vi "test control disable.vi"(0 "Robot Mode":T3(ring), 1 "Test Mode":T2(ring)) -> (2 "Display Test?":bool, 3 "Why Disabled?":string, 4 "Disabled":T1(ring))   [LabVIEW 2015]
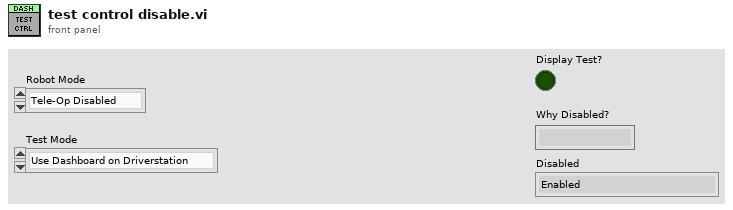
[diagram p1: front panel]
types:
  T1 = enum8{"Enabled", "Disabled", "Disabled and Grayed Out"}
  T2 = enum32{"Use Dashboard on Driverstation", "Use Programmer's Laptop"}
  T3 = enum8{"Tele-Op Disabled", "Tele-Op Enabled", "Auto Disabled", "Auto Enabled", "Test Disabled", "Test Enabled", "Disconnected", "No Code", "E-Stop"}
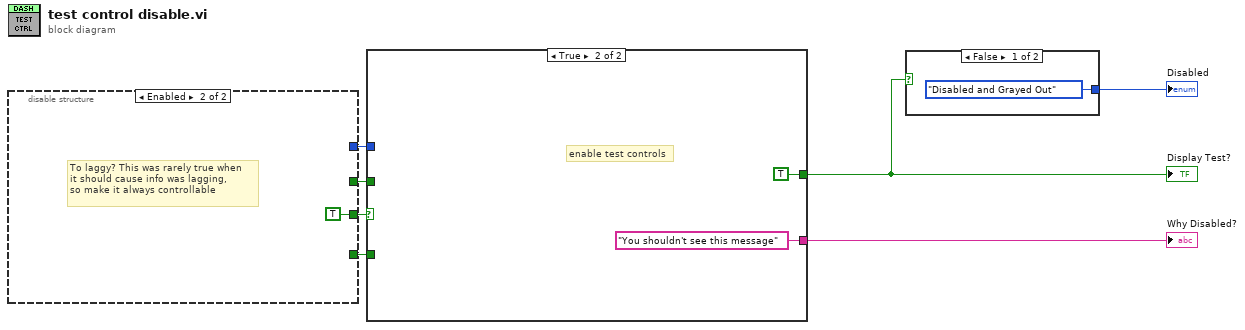
[diagram p0: block diagram]
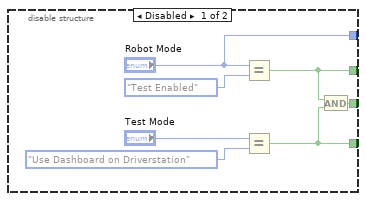
[diagram p2: hidden frame]
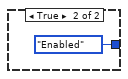
[diagram p3: hidden frame]
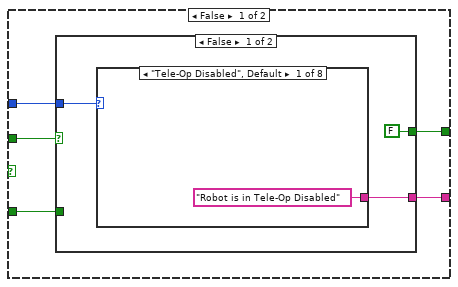
[diagram p4: hidden frame]
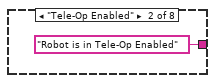
[diagram p5: hidden frame]
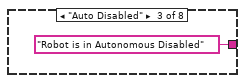
[diagram p6: hidden frame]
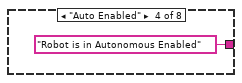
[diagram p7: hidden frame]
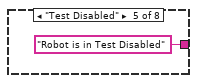
[diagram p8: hidden frame]
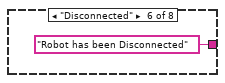
[diagram p9: hidden frame]
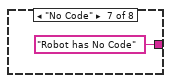
[diagram p10: hidden frame]
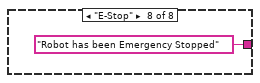
[diagram p11: hidden frame]
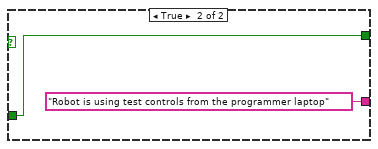
[diagram p12: hidden frame]
diagram:
  n1 = disable-structure shown="Enabled" {
    disable-tunnel: [w11 TRUE] -> w7
    disable-tunnel: [w10 _] -> w5
    disable-tunnel: [w9 _] -> w4
    disable-tunnel: ["Robot Mode" _] -> w3
    frame Disabled {
      n2 = Equal?(x="Robot Mode", y=T3."Test Enabled") -> (x = y?=w10:bool)
      n3 = Equal?(x="Test Mode", y=T2."Use Dashboard on Driverstation") -> (x = y?=w9:bool)
      n4 = And(x=w10, y=w9) -> (x .and. y?=w11:bool)
    }
    frame Enabled {
      # "To laggy? This was rarely true when\nit should cause info was lagging,\nso make it always controllable"
    }
  }
  n5 = case shown="True" w7 {
    tunnel: [w18 TRUE] -> w2
    tunnel: [w17 "You shouldn't see this message" ("Why Disabled?")] -> w6
    tunnel: w5 -> [w20 _]
    tunnel: w4 -> [w19 _]
    tunnel: w3 -> [w16 _]
    frame False {
      n6 = case shown="False" w20 {
        tunnel: w19 -> [_ w32]
        tunnel: [FALSE w32] -> w18
        tunnel: [w21 "Robot is using test controls from the programmer laptop" ("Why Disabled?")] -> w17
        tunnel: w16 -> [w22 _]
        frame False {
          n7 = case shown="\"Tele-Op Disabled\", Default" w22 {
            tunnel: ["Robot is in Tele-Op Disabled" ("Why Disabled?") "Robot is in Tele-Op Enabled" ("Why Disabled?") "Robot is in Autonomous Disabled" ("Why Disabled?") "Robot is in Autonomous Enabled" ("Why Disabled?") "Robot is in Test Disabled" ("Why Disabled?") "Robot has been Disconnected" ("Why Disabled?") "Robot has No Code" ("Why Disabled?") "Robot has been Emergency Stopped" ("Why Disabled?")] -> w21
            frame "Tele-Op Disabled", Default {
            }
            frame "Tele-Op Enabled" {
            }
            frame "Auto Disabled" {
            }
            frame "Auto Enabled" {
            }
            frame "Test Disabled" {
            }
            frame "Disconnected" {
            }
            frame "No Code" {
            }
            frame "E-Stop" {
            }
          }
        }
        frame True {
        }
      }
    }
    frame True {
      # "enable test controls"
    }
  }
  "Display Test?" <- w2
  "Why Disabled?" <- w6
  n8 = case shown="False" w2 {
    tunnel: [T1."Disabled and Grayed Out" ("Disabled") T1."Enabled" ("Disabled")] -> w1
    frame False {
    }
    frame True {
    }
  }
  "Disabled" <- w1
